vi "Lead Screw Practice.vi"() -> ()   [LabVIEW 2012]
uses:
  <vilib>/Rock Robotics/WPI/Joystick/WPI_JoystickGetSetRefNum.vi
panel:
  out "Calculated Lead Screw Angle":dbl
  in  "Encoder Error Offset":dbl
  out "Encoder Lead Screw Angle":dbl
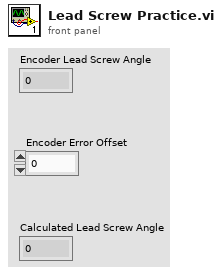
[diagram p1: front panel]
types:
  T1 = typedef "WPI_EncoderDevRef.ctl" = cluster{"DevStatus":errorcluster, "EncoderIndex":T2, "CounterIndex":T3, "DistancePerCount":dbl, "Decoding Type":T4}
  T2 = typedef "FPGA_EncoderIdx.ctl" = enum8{"Enc 0", "Enc 1", "Enc 2", "Enc 3", "Invalid"}
  T3 = typedef "FPGA_CounterCtrSystemIndex.ctl" = enum8{"Ctr 0", "Ctr 1", "Ctr 2", "Ctr 3", "Ctr 4", "Ctr 5", "Ctr 6", "Ctr 7", "Invalid"}
  T4 = typedef "WPI_EncoderType.ctl" = enum16{"1x", "2x", "4x"}
  T5 = typedef "WPI_DigitalInputDevRef.ctl" = cluster{"DevStatus":errorcluster, "DIO Channel":T6, "Digital Module":T7}
  T6 = typedef "FPGA_DIOChannel.ctl" = enum8{"DIO 1", "DIO 2", "DIO 3", "DIO 4", "DIO 5", "DIO 6", "DIO 7", "DIO 8", "DIO 9", "DIO 10", "DIO 11", "DIO 12", "DIO 13", "DIO 14", "Invalid"}
  T7 = typedef "FPGA_TypedefDigitalModule.ctl" = enum16{"Digital Module 1", "Digital Module 2"}
  T8 = typedef "WPI_JoystickDevRef.ctl" = cluster{"Device":T9}
  T9 = typedef "WPI_JoystickDeviceEnum.ctl" = enum16{"USB 1", "USB 2", "USB 3", "USB 4", "Kinect 1", "Kinect 2"}
  T10 = cluster{"axis 1 (x)":dbl, "axis 2 (y)":dbl, "axis 3 (throttle)":dbl, "axis 4":dbl, "axis 5":dbl, "axis 6":dbl}
  T11 = typedef "WPI_MotorControlDeviceRef.ctl" = cluster{"DeviceStatus":errorcluster, "Type":enum16{"PWM", "CAN"}, "PWM":cluster{"Digital Module":T7, "PWM Channel":T12, "DeadBand":T13}, "CAN":cluster{"Device Number":u8, "Control Mode":T14, "Semaphore":T15, "Max Vout":dbl}, "Invert":bool, "TransformRef":T16, "InvTransformRef":T16}
  T12 = typedef "FPGA_DIOPWMChannel.ctl" = enum8{"PWM 1", "PWM 2", "PWM 3", "PWM 4", "PWM 5", "PWM 6", "PWM 7", "PWM 8", "PWM 9", "PWM 10", "Invalid"}
  T13 = typedef "WPI_PWMDeadband.ctl" = cluster{"Name":string, "maxPositivePwm":i32, "minPositivePwm":i32, "centerPwm":i32, "maxNegativePwm":i32, "minNegativePwm":i32, "angularRange":u16}
  T14 = typedef "WPI_CANJaguar_ControlMode.ctl" = enum8{"Percent VBus", "Current", "Speed", "Position", "Voltage"}
  T15 = typedef "Semaphore RefNum" = refnum<k1>
  T16 = typedef "WPI_PWMTransform_ConPane.ctl" = refnum<vi>
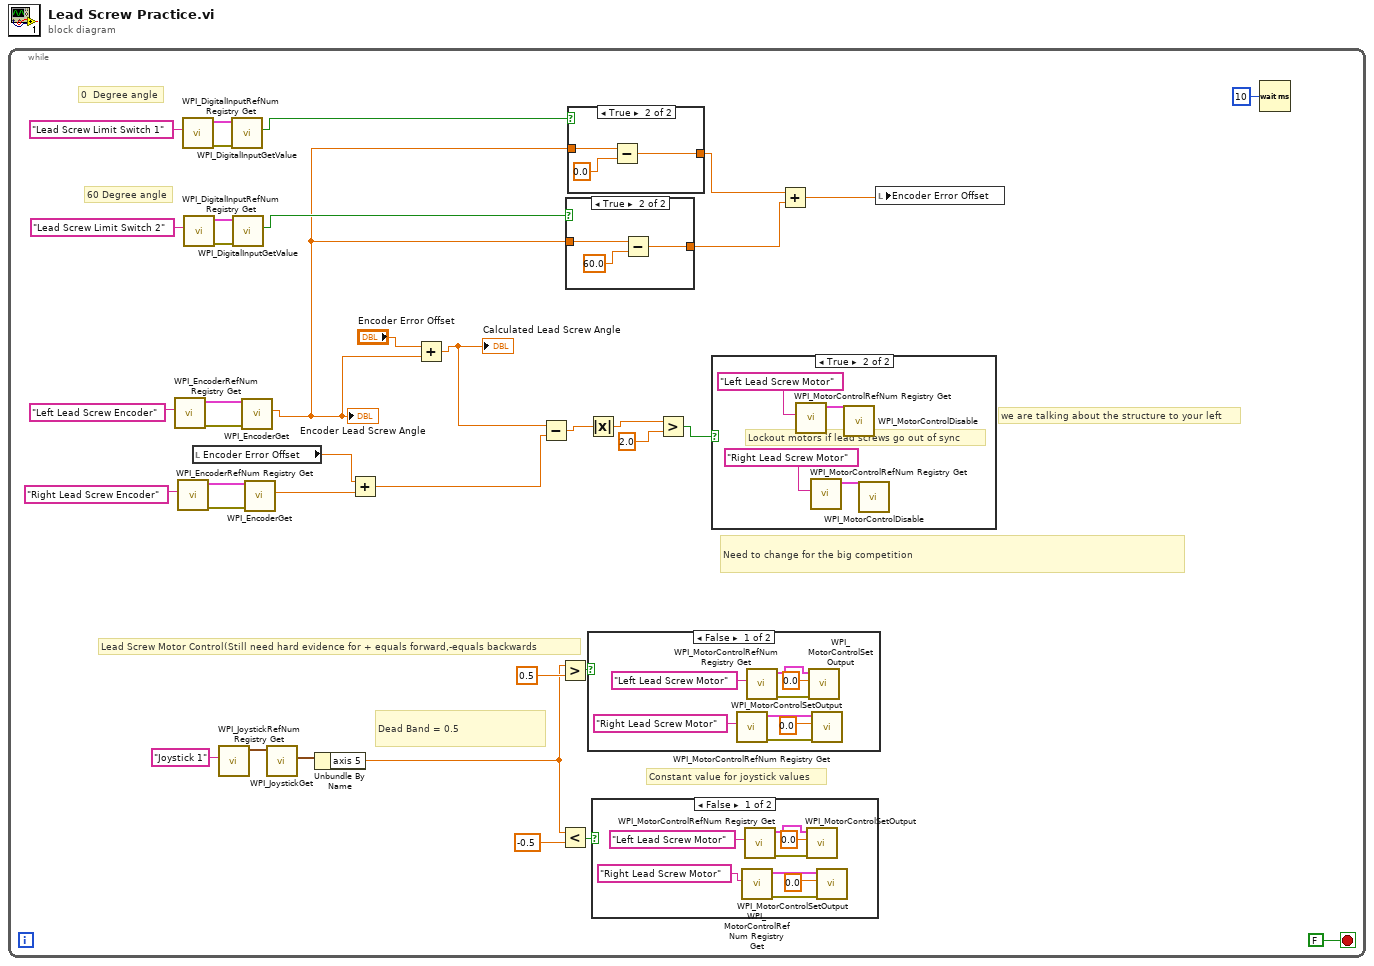
[diagram p0: block diagram]
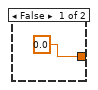
[diagram p3: hidden frame]
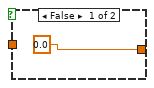
[diagram p4: hidden frame]
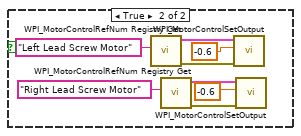
[diagram p5: hidden frame]
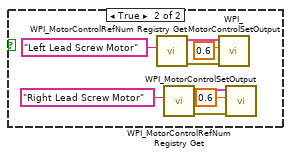
[diagram p6: hidden frame]
diagram:
  n1 = while {
    stop <- FALSE stop-if-true
    # "we are talking about the structure to your left"
    # "Need to change for the big competition"
    # "60 Degree angle"
    # "0  Degree angle"
    # "Dead Band = 0.5"
    # "Constant value for joystick values"
    # "Lead Screw Motor Control(Still need hard evidence for + equals forward,-equals backwards"
    n2 = call <vilib>:"WPI_EncoderRefNum Registry Get.vi"("refnum name"="Left Lead Screw Encoder") -> ("error out"=w19:errorcluster, "EncoderDevRef"=w20:T1)  [unwired: 9 in]
    n3 = call <vilib>:"WPI_EncoderRefNum Registry Get.vi"("refnum name"="Right Lead Screw Encoder") -> ("error out"=w11:errorcluster, "EncoderDevRef"=w12:T1)  [unwired: 9 in]
    n4 = call <vilib>:"WPI_DigitalInputRefNum Registry Get.vi"("refnum name"="Lead Screw Limit Switch 1") -> ("error out"=w36:errorcluster, "DigitalInputDevRef"=w35:T5)  [unwired: 9 in]
    n5 = call <vilib>:"WPI_DigitalInputRefNum Registry Get.vi"("refnum name"="Lead Screw Limit Switch 2") -> ("error out"=w33:errorcluster, "DigitalInputDevRef"=w32:T5)  [unwired: 9 in]
    n6 = local read "Encoder Error Offset"() -> (w9:dbl)
    n7 = call <vilib>:"WPI_JoystickRefNum Registry Get.vi"("refnum name"="Joystick 1") -> ("JoystickDevRef"=w30:T8)  [unwired: 9 in, 1 out]
    n8 = call <vilib>:"WPI_DigitalInputGetValue.vi"("error in (no error)"=w36, "DigitalInputDevRef"=w35) -> ("Value"=w23:bool)  [unwired: 7 in, 2 out]
    n9 = call <vilib>:"WPI_DigitalInputGetValue.vi"("error in (no error)"=w33, "DigitalInputDevRef"=w32) -> ("Value"=w22:bool)  [unwired: 7 in, 2 out]
    n10 = call <vilib>:"WPI_EncoderGet.vi"("error in (no error)"=w19, "EncoderDevRef"=w20) -> ("Distance"=w15:dbl)  [unwired: 4 in, 5 out]
    "Encoder Lead Screw Angle" <- w15
    n11 = call <vilib>:"WPI_EncoderGet.vi"("error in (no error)"=w11, "EncoderDevRef"=w12) -> ("Distance"=w10:dbl)  [unwired: 4 in, 5 out]
    n12 = call <vilib>:"WPI_JoystickGet.vi"("JoystickDevRef"=w30) -> ("Axes"=w29:T10)  [unwired: 4 in, 2 out]
    n13 = Unbundle By Name(w29) -> ("axis 5"=w24:dbl)
    n14 = Add(x=w9, y=w10) -> (x+y=w8:dbl)
    n15 = Add(x="Encoder Error Offset", y=w15) -> (x+y=w7:dbl)
    "Calculated Lead Screw Angle" <- w7
    n16 = Subtract(x=w7, y=w8) -> (x-y=w6:dbl)
    n17 = Greater?(x=w24, y=0.5) -> (0:w27:bool)
    n18 = Less?(x=w24, y=-0.5) -> (x < y?=w25:bool)
    n19 = case shown="True" w22 {
      tunnel: w15 -> [_ w44]
      tunnel: [0.0 w43] -> w17
      frame False {
      }
      frame True {
        n20 = Subtract(x=w44, y=60.0) -> (x-y=w43:dbl)
      }
    }
    n21 = case shown="True" w23 {
      tunnel: w15 -> [_ w49]
      tunnel: [0.0 w47] -> w18
      frame False {
      }
      frame True {
        n22 = Subtract(x=w49, y=0.0) -> (x-y=w47:dbl)
      }
    }
    n23 = Absolute Value(x=w6) -> (abs(x)=w5:dbl)
    n24 = case shown="False" w27 {
      frame False {
        n25 = call <vilib>:"WPI_MotorControlRefNum Registry Get.vi"("refnum name"="Right Lead Screw Motor") -> ("error out"=w69:errorcluster, "MotorControlDevRef"=w68:T11)  [unwired: 9 in]
        n26 = call <vilib>:"WPI_MotorControlRefNum Registry Get.vi"("refnum name"="Left Lead Screw Motor") -> ("error out"=w72:errorcluster, "MotorControlDevRef"=w66:T11)  [unwired: 9 in]
        n27 = call <vilib>:"WPI_MotorControlSetOutput.vi"("error in (no error)"=w72, "Output"=0.0, "MotorControlDevRef"=w66) -> ()  [unwired: 6 in, 3 out]
        n28 = call <vilib>:"WPI_MotorControlSetOutput.vi"("error in (no error)"=w69, "Output"=0.0, "MotorControlDevRef"=w68) -> ()  [unwired: 6 in, 3 out]
      }
      frame True {
        n29 = call <vilib>:"WPI_MotorControlRefNum Registry Get.vi"("refnum name"="Left Lead Screw Motor") -> ("error out"=w80:errorcluster, "MotorControlDevRef"=w79:T11)  [unwired: 9 in]
        n30 = call <vilib>:"WPI_MotorControlRefNum Registry Get.vi"("refnum name"="Right Lead Screw Motor") -> ("error out"=w76:errorcluster, "MotorControlDevRef"=w75:T11)  [unwired: 9 in]
        n31 = call <vilib>:"WPI_MotorControlSetOutput.vi"("error in (no error)"=w80, "Output"=0.6, "MotorControlDevRef"=w79) -> ()  [unwired: 6 in, 3 out]
        n32 = call <vilib>:"WPI_MotorControlSetOutput.vi"("error in (no error)"=w76, "Output"=0.6, "MotorControlDevRef"=w75) -> ()  [unwired: 6 in, 3 out]
      }
    }
    n33 = case shown="False" w25 {
      frame False {
        n34 = call <vilib>:"WPI_MotorControlRefNum Registry Get.vi"("refnum name"="Right Lead Screw Motor") -> ("error out"=w54:errorcluster, "MotorControlDevRef"=w53:T11)  [unwired: 9 in]
        n35 = call <vilib>:"WPI_MotorControlRefNum Registry Get.vi"("refnum name"="Left Lead Screw Motor") -> ("error out"=w56:errorcluster, "MotorControlDevRef"=w51:T11)  [unwired: 9 in]
        n36 = call <vilib>:"WPI_MotorControlSetOutput.vi"("error in (no error)"=w56, "Output"=0.0, "MotorControlDevRef"=w51) -> ()  [unwired: 6 in, 3 out]
        n37 = call <vilib>:"WPI_MotorControlSetOutput.vi"("error in (no error)"=w54, "Output"=0.0, "MotorControlDevRef"=w53) -> ()  [unwired: 6 in, 3 out]
      }
      frame True {
        n38 = call <vilib>:"WPI_MotorControlRefNum Registry Get.vi"("refnum name"="Left Lead Screw Motor") -> ("error out"=w64:errorcluster, "MotorControlDevRef"=w63:T11)  [unwired: 9 in]
        n39 = call <vilib>:"WPI_MotorControlRefNum Registry Get.vi"("refnum name"="Right Lead Screw Motor") -> ("error out"=w60:errorcluster, "MotorControlDevRef"=w59:T11)  [unwired: 9 in]
        n40 = call <vilib>:"WPI_MotorControlSetOutput.vi"("error in (no error)"=w64, "Output"=-0.6, "MotorControlDevRef"=w63) -> ()  [unwired: 6 in, 3 out]
        n41 = call <vilib>:"WPI_MotorControlSetOutput.vi"("error in (no error)"=w60, "Output"=-0.6, "MotorControlDevRef"=w59) -> ()  [unwired: 6 in, 3 out]
      }
    }
    n42 = Greater?(x=w5, y=2.0) -> (0:w3:bool)
    n43 = case shown="True" w3 {
      frame False {
      }
      frame True {
        # "Lockout motors if lead screws go out of sync"
        n44 = call <vilib>:"WPI_MotorControlRefNum Registry Get.vi"("refnum name"="Left Lead Screw Motor") -> ("MotorControlDevRef"=w40:T11)  [unwired: 9 in, 1 out]
        n45 = call <vilib>:"WPI_MotorControlRefNum Registry Get.vi"("refnum name"="Right Lead Screw Motor") -> ("MotorControlDevRef"=w38:T11)  [unwired: 9 in, 1 out]
        n46 = call <vilib>:"WPI_MotorControlDisable.vi"("MotorControlDevRef"=w40) -> ()  [unwired: 9 in, 2 out]
        n47 = call <vilib>:"WPI_MotorControlDisable.vi"("MotorControlDevRef"=w38) -> ()  [unwired: 9 in, 2 out]
      }
    }
    n48 = Add(x=w18, y=w17) -> (x+y=w16:dbl)
    n49 = local write "Encoder Error Offset"(w16) -> ()
    n50 = Wait (ms)(milliseconds to wait=u32 10) -> ()  [unwired: 1 out]
  }
